vi "Scan Larvae Contour (SubVI).vi"(0 "Data In":u8=255, 1 "Input Valid?":bool, 3 "X Start":u16, 4 "Y Start":u16, 6 "Max. Scan Cycles":u32=40000) -> (13 "Ready for Input?":bool, 14 "Boundary Point XY":u32, 15 "Boundary Valid?":bool, 16 "Scan End?":bool, 19 "Total ClkCyls":u32)   [LabVIEW 2015]
uses:
  Controls (FPGA)/Larvae Contour States DRAM.ctl
  Controls (FPGA)/Contour Scan.ctl
  <vilib>/rvi/Emulation/niFpgaProcessEmulError.vi
  <vilib>/rvi/Emulation/niFpgaEmulationIsFPGAContextNoSignature.vi
  <vilib>/rvi/Emulation/niFpgaSctlEmulationGetInTimedLoop.vi
  <vilib>/rvi/errors/niFpgaSetErrorForExecOnDevCompSimple.vi
  <vilib>/rvi/eio/common/nirviEmuReportErrorAndStop.vi
  <vilib>/rvi/DataTransferAndStorage/Container/Common/niFpgaContainerGetUniqueNameForEmu.vi
  <vilib>/rvi/FIFO/Fifo_Resource/nirvififoEmulationSetSize.vi
  <vilib>/rvi/FIFO/Fifo_Resource/nirviFifoEmulationQueueMgr.vi
  <instcachedir>/0/nirviFifoEmulationQueueMgr_E5CAEC123FF24DC58D834DCA3CDAA9B5.lvgen/nirviFifoEmulationQueueMgr_E5CAEC123FF24DC58D834DCA3CDAA9B5_001.vi
  <vilib>/Utility/error.llb/Clear Errors.vi
  <vilib>/rvi/FIFO/Fifo_Resource/nirvififoEmulationCreateLock.vi
  <vilib>/rvi/FIFO/Fifo_Resource/nirvififoEmulationObtainLock.vi
  <vilib>/rvi/FIFO/Fifo_Resource/nirvififoEmulationReleaseLock.vi
  <vilib>/rvi/occurrence/nirviWaitOnOccurrenceBase.vi
  <vilib>/rvi/errors/nirviReportUnexpectedCaseInternalError.vi
  <vilib>/rvi/errors/nirviReportUnexpectedCaseInternalError (U32).vi
  <instcachedir>/0/nirviFifoEmulationQueueMgr_E5CAEC123FF24DC58D834DCA3CDAA9B5.lvgen/nirviFifoEmulationQueueMgr_E5CAEC123FF24DC58D834DCA3CDAA9B5_004.vi
  <vilib>/rvi/FIFO/Fifo_Resource/nirvififoEmulationDetermineInputValidOut.vi
  <vilib>/rvi/DataTransferAndStorage/Container/XNode/niFpgaContainer.xnode
  <vilib>/rvi/FIFO/Fifo_Resource/nirvififoEmulationRead.vi
  <vilib>/rvi/FIFO/Fifo_Resource/nirvififoEmulationWrite.vi
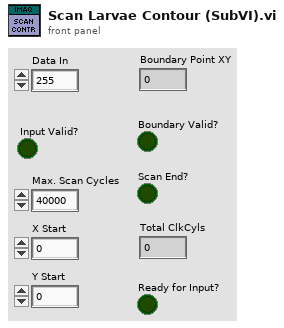
[diagram p1: front panel]
types:
  T1 = typedef "Contour Scan.ctl" = cluster{"Next Address":fxp<+,24,24>, "Next X":fxp<+,12,12>, "Next Y":fxp<+,12,12>, "Current Address":fxp<+,24,24>, "Current X":fxp<+,12,12>, "Current Y":fxp<+,12,12>, "Scan Count":u32}
  T2 = typedef "Larvae Contour States DRAM.ctl" = enum8{"Intialize", "Loop Condition", "Pixel 1", "Pixel 2", "Pixel 3", "Pixel 4", "Pixel 5", "Pixel 6", "Pixel 7", "Pixel 8", "Retrieve Data", "End of Scan"}
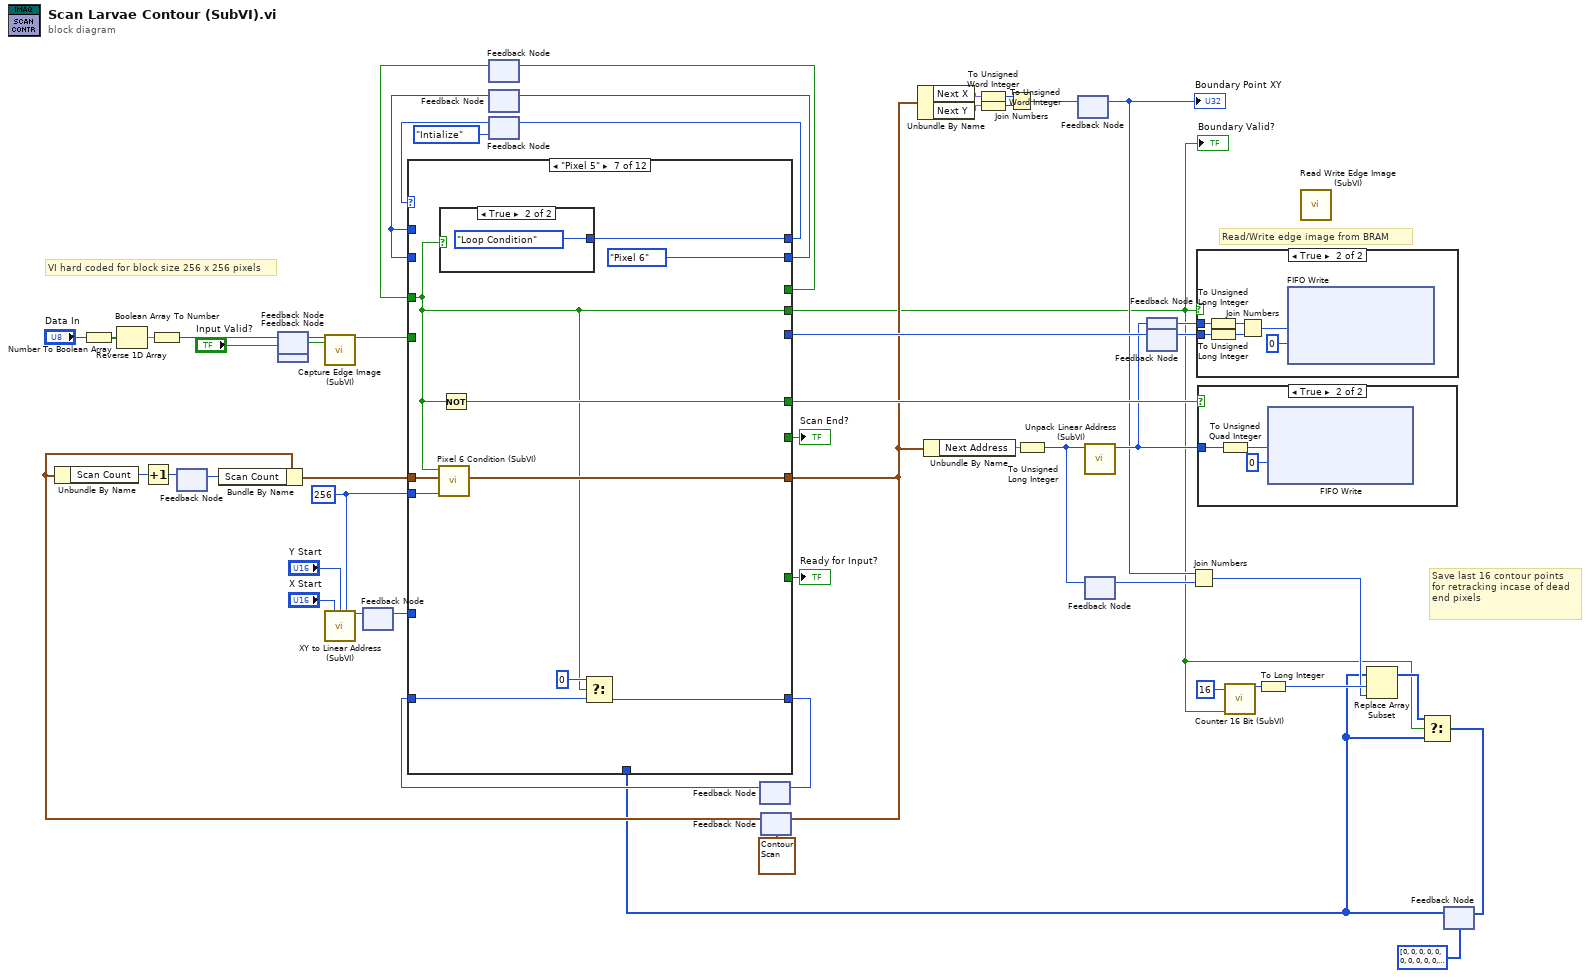
[diagram p0: block diagram]
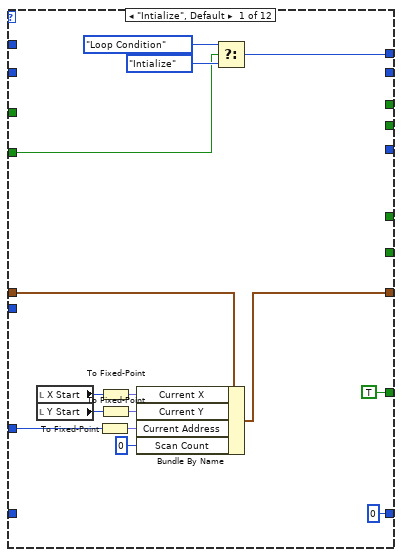
[diagram p4: hidden frame]
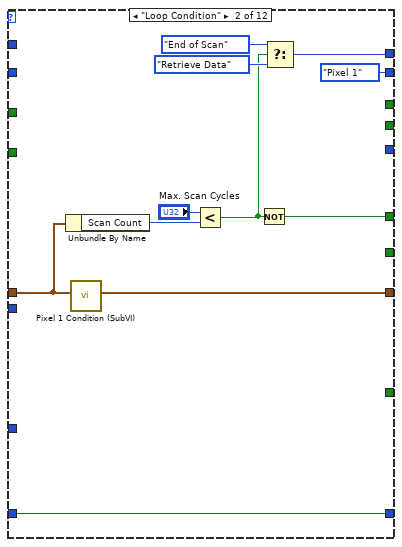
[diagram p5: hidden frame]
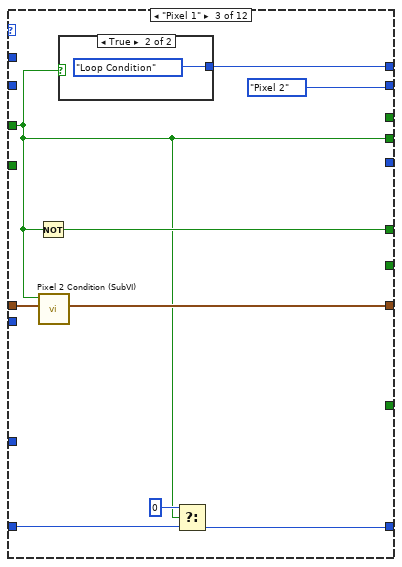
[diagram p6: hidden frame]
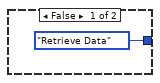
[diagram p7: hidden frame]
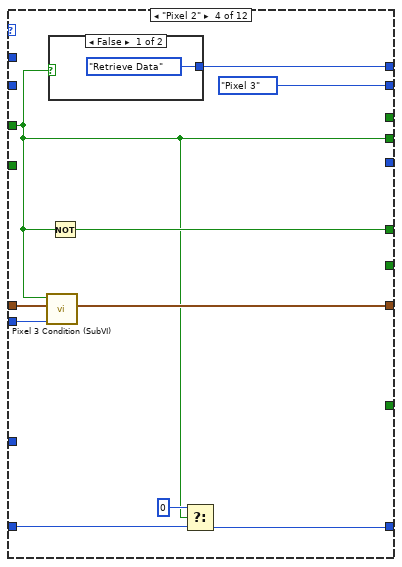
[diagram p8: hidden frame]
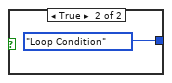
[diagram p9: hidden frame]
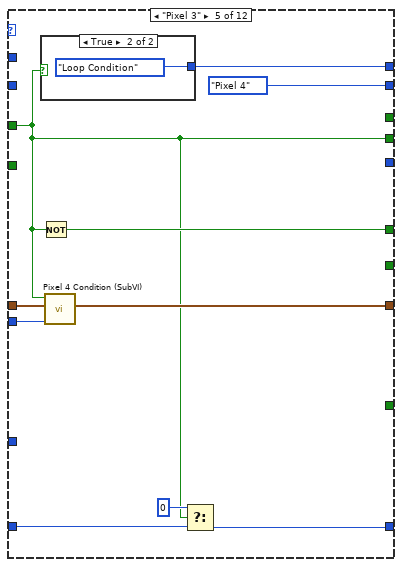
[diagram p10: hidden frame]
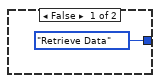
[diagram p11: hidden frame]
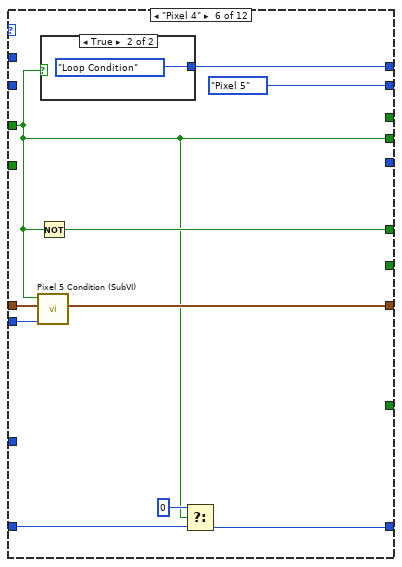
[diagram p12: hidden frame]
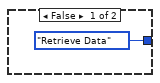
[diagram p13: hidden frame]
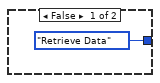
[diagram p14: hidden frame]
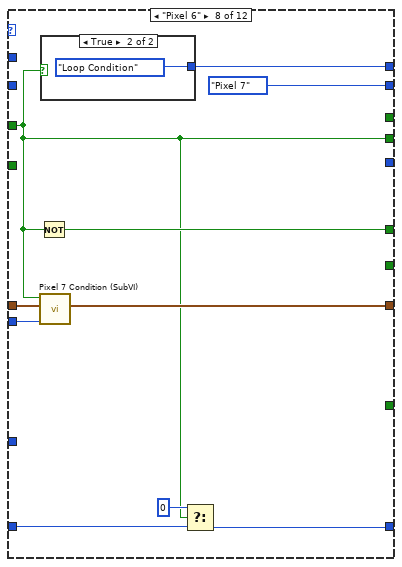
[diagram p15: hidden frame]
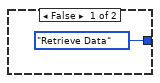
[diagram p16: hidden frame]
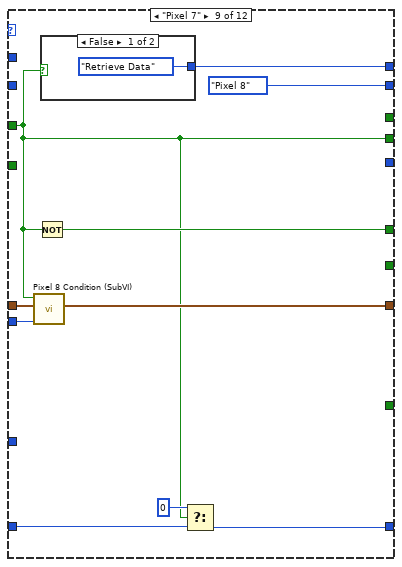
[diagram p17: hidden frame]
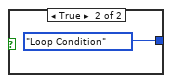
[diagram p18: hidden frame]
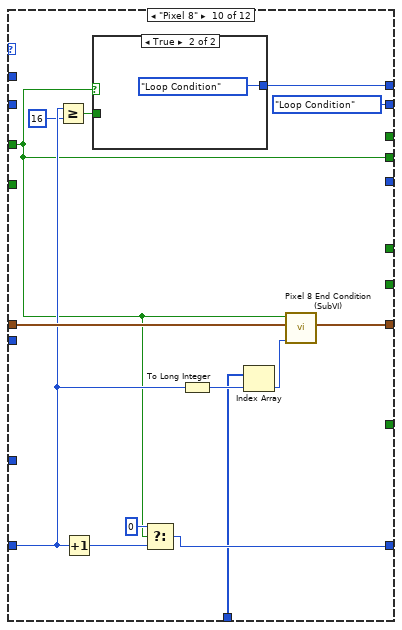
[diagram p19: hidden frame]
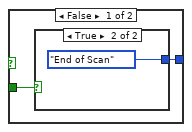
[diagram p20: hidden frame]
diagram:
  w23 = u16 256 ("Image Width")
  # "Save last 16 contour points for retracking incase of dead end pixels"
  # "VI hard coded for block size 256 x 256 pixels"
  # "Read/Write edge image from BRAM"
  n1 = Number To Boolean Array(number="Data In") -> (Boolean array=w21:bool[])
  n2 = Reverse 1D Array(array=w21) -> (reversed array=w22:bool[])
  n3 = Boolean Array To Number(Boolean array=w22) -> (number=w19:u8)
  n4 = feedback #1() -> (w30:u32)  [unwired: 1 in]
  n5 = feedback-in #2(w19) -> ()
  n6 = feedback #2() -> (w44:u8)  [unwired: 1 in]
  n7 = feedback-in #3("Input Valid?") -> ()
  n8 = feedback #3() -> (w43:bool)  [unwired: 1 in]
  n9 = call "Capture Edge Image (SubVI).vi"("Data In"=w44, "Data Valid?"=w43) -> ("Capture End?"=w42:bool)  [unwired: 17 in]
  n10 = call "XY to Linear Address (SubVI).vi"("X"="X Start", "Y"="Y Start", "Image Width"=w23) -> ("Linear Address"=w41:u32)  [unwired: 12 in]
  n11 = feedback-in #4(w41) -> ()
  n12 = feedback #4() -> (w40:u32)  [unwired: 1 in]
  n13 = feedback #5() -> (w17:bool)  [unwired: 1 in]
  n14 = feedback #6() -> (w50:T2)  [unwired: 1 in]
  n15 = feedback #7(Larvae_Contour_States_DRAM."Intialize") -> (w52:T2)
  n16 = feedback #8() -> (w12:u8)  [unwired: 1 in]
  n17 = feedback #9(T1 {"Next Address"=0.0, "Next X"=0.0, "Next Y"=0.0, "Current Address"=0.0, "Current X"=0.0, "Current Y"=0.0, "Scan Count"=0}) -> (w36:T1)
  n18 = Unbundle By Name(w36) -> ("Scan Count"=w35:u32)
  n19 = Increment(x=w35) -> (x+1=w34:u32)
  n20 = feedback-in #1(w34) -> ()
  n21 = Bundle By Name(cluster=w36, "Scan Count"=w30) -> (w37:T1)
  n22 = feedback #10() -> (w2:u32)  [unwired: 1 in]
  "Boundary Point XY" <- w2
  n23 = feedback #11() -> (w3:u32)  [unwired: 1 in]
  n24 = feedback #12() -> (w47:u32)  [unwired: 1 in]
  n25 = feedback #13() -> (w48:u8)  [unwired: 1 in]
  n26 = Join Numbers(hi=w2, lo=w3) -> ((hi.lo)=w8:u64)
  n27 = call "Read Write Edge Image (SubVI).vi"() -> ()  [unwired: 12 in]
  n28 = feedback #14(u64[] [0, 0, 0, 0, 0, 0, 0, 0, 0, 0, 0, 0, 0, 0, 0, 0]) -> (w6:u64[])
  n29 = case shown="\"Pixel 5\"" w52 {
    tunnel: [w68 w80 w89 w99 w111 w123 w135 w147 w159 w176 w198 Larvae_Contour_States_DRAM."Intialize" ("f")] -> w54
    tunnel: [_ _ w81 w92 w104 w116 w128 w140 w152 w166 _ _] -> w1
    tunnel: [_ _ _ _ _ _ _ _ _ _ _ TRUE] -> w27
    tunnel: w17 -> [_ _ w81 w92 w104 w116 w128 w140 w152 w166 _ _]
    tunnel: [_ w76 w88 w101 w113 w125 w137 w149 w161 _ _ _] -> w46
    tunnel: [_ Larvae_Contour_States_DRAM."Pixel 1" ("f") Larvae_Contour_States_DRAM."Pixel 2" ("f") Larvae_Contour_States_DRAM."Pixel 3" ("f") Larvae_Contour_States_DRAM."Pixel 4" ("f") Larvae_Contour_States_DRAM."Pixel 5" ("f") Larvae_Contour_States_DRAM."Pixel 6" ("f") Larvae_Contour_States_DRAM."Pixel 7" ("f") Larvae_Contour_States_DRAM."Pixel 8" ("f") Larvae_Contour_States_DRAM."Loop Condition" ("f") w197 _] -> w51
    tunnel: w50 -> [_ _ _ _ _ _ _ _ _ _ w199 _]
    tunnel: [_ _ _ _ _ _ _ _ _ _ w201 _] -> w5
    tunnel: w50 -> [_ _ _ _ _ _ _ _ _ _ w197 _]
    tunnel: [_ _ _ _ _ _ _ _ _ _ w193 _] -> w49
    tunnel: w42 -> [w66 _ _ _ _ _ _ _ _ _ _ _]
    tunnel: w40 -> [w64 _ _ _ _ _ _ _ _ _ _ _]
    tunnel: w37 -> [w65 w72 w86 w98 w109 w122 w134 w146 w157 w175 w186 w204]
    tunnel: [w62 w75 w85 w97 w110 w121 w133 w145 w158 w174 w186 w204] -> w26
    tunnel: w23 -> [_ _ _ w96 w108 w120 w132 w144 w156 _ _ _]
    tunnel: [TRUE _ _ _ _ _ _ _ _ _ _ _] -> w18
    tunnel: w6 -> [_ _ _ _ _ _ _ _ _ w164 _ _]
    tunnel: [u8 0 ("Scan Count") w70 w83 w94 w106 w118 w130 w142 w154 w171 w183 w202] -> w13
    tunnel: w12 -> [_ w70 w84 w95 w107 w119 w131 w143 w155 w169 w183 w202]
    frame "Intialize", Default {
      n30 = local read "X Start"() -> (w58:u16)
      n31 = local read "Y Start"() -> (w57:u16)
      n32 = To Fixed-Point(number=w64) -> (fixed-point=w59:fxp<+,24,24>)  [unwired: 1 in]
      n33 = To Fixed-Point(number=w58) -> (fixed-point=w61:fxp<+,12,12>)  [unwired: 1 in]
      n34 = To Fixed-Point(number=w57) -> (fixed-point=w60:fxp<+,12,12>)  [unwired: 1 in]
      n35 = Bundle By Name(cluster=w65, "Current X"=w61, "Current Y"=w60, "Current Address"=w59, "Scan Count"=u32 0) -> (w62:T1)
      n36 = Select(t=Larvae_Contour_States_DRAM."Loop Condition", s=w66, f=Larvae_Contour_States_DRAM."Intialize") -> (s? t:f=w68:T2)
    }
    frame "Loop Condition" {
      n37 = Unbundle By Name(w72) -> ("Scan Count"=w74:u32)
      n38 = call "Pixel 1 Condition (SubVI).vi"("Contour Scan in"=w72) -> ("Contour Scan out"=w75:T1)  [unwired: 10 in]
      n39 = Less?(x="Max. Scan Cycles", y=w74) -> (x < y?=w73:bool)
      n40 = Not(x=w73) -> (.not. x?=w76:bool)
      n41 = Select(t=Larvae_Contour_States_DRAM."End of Scan", s=w73, f=Larvae_Contour_States_DRAM."Retrieve Data") -> (s? t:f=w80:T2)
    }
    frame "Pixel 1" {
      n42 = Not(x=w81) -> (.not. x?=w88:bool)
      n43 = call "Pixel 2 Condition (SubVI).vi"("Contour Scan in"=w86, "Fnd?"=w81) -> ("Contour Scan out"=w85:T1)  [unwired: 9 in]
      n44 = case shown="True" w81 {
        tunnel: [Larvae_Contour_States_DRAM."Retrieve Data" ("f") Larvae_Contour_States_DRAM."Loop Condition" ("f")] -> w89
        frame False {
        }
        frame True {
        }
      }
      n45 = Select(t=u8 0, s=w81, f=w84) -> (s? t:f=w83:u8)
    }
    frame "Pixel 2" {
      n46 = call "Pixel 3 Condition (SubVI).vi"("Image Width"=w96, "Contour Scan in"=w98, "Fnd?"=w92) -> ("Contour Scan out"=w97:T1)  [unwired: 8 in]
      n47 = case shown="False" w92 {
        tunnel: [Larvae_Contour_States_DRAM."Retrieve Data" ("f") Larvae_Contour_States_DRAM."Loop Condition" ("f")] -> w99
        frame False {
        }
        frame True {
        }
      }
      n48 = Not(x=w92) -> (.not. x?=w101:bool)
      n49 = Select(t=u8 0, s=w92, f=w95) -> (s? t:f=w94:u8)
    }
    frame "Pixel 3" {
      n50 = case shown="True" w104 {
        tunnel: [Larvae_Contour_States_DRAM."Retrieve Data" ("f") Larvae_Contour_States_DRAM."Loop Condition" ("f")] -> w111
        frame False {
        }
        frame True {
        }
      }
      n51 = Not(x=w104) -> (.not. x?=w113:bool)
      n52 = call "Pixel 4 Condition (SubVI).vi"("Image Width"=w108, "Contour Scan in"=w109, "Fnd?"=w104) -> ("Contour Scan out"=w110:T1)  [unwired: 8 in]
      n53 = Select(t=u8 0, s=w104, f=w107) -> (s? t:f=w106:u8)
    }
    frame "Pixel 4" {
      n54 = call "Pixel 5 Condition (SubVI).vi"("Image Width"=w120, "Contour Scan in"=w122, "Fnd?"=w116) -> ("Contour Scan out"=w121:T1)  [unwired: 8 in]
      n55 = Not(x=w116) -> (.not. x?=w125:bool)
      n56 = case shown="True" w116 {
        tunnel: [Larvae_Contour_States_DRAM."Retrieve Data" ("f") Larvae_Contour_States_DRAM."Loop Condition" ("f")] -> w123
        frame False {
        }
        frame True {
        }
      }
      n57 = Select(t=u8 0, s=w116, f=w119) -> (s? t:f=w118:u8)
    }
    frame "Pixel 5" {
      n58 = call "Pixel 6 Condition (SubVI).vi"("Image Width"=w132, "Contour Scan in"=w134, "Fnd?"=w128) -> ("Contour Scan out"=w133:T1)  [unwired: 8 in]
      n59 = case shown="True" w128 {
        tunnel: [Larvae_Contour_States_DRAM."Retrieve Data" ("f") Larvae_Contour_States_DRAM."Loop Condition" ("f")] -> w135
        frame False {
        }
        frame True {
        }
      }
      n60 = Not(x=w128) -> (.not. x?=w137:bool)
      n61 = Select(t=u8 0, s=w128, f=w131) -> (s? t:f=w130:u8)
    }
    frame "Pixel 6" {
      n62 = Not(x=w140) -> (.not. x?=w149:bool)
      n63 = call "Pixel 7 Condition (SubVI).vi"("Image Width"=w144, "Contour Scan in"=w146, "Fnd?"=w140) -> ("Contour Scan out"=w145:T1)  [unwired: 8 in]
      n64 = case shown="True" w140 {
        tunnel: [Larvae_Contour_States_DRAM."Retrieve Data" ("f") Larvae_Contour_States_DRAM."Loop Condition" ("f")] -> w147
        frame False {
        }
        frame True {
        }
      }
      n65 = Select(t=u8 0, s=w140, f=w143) -> (s? t:f=w142:u8)
    }
    frame "Pixel 7" {
      n66 = call "Pixel 8 Condition (SubVI).vi"("Image Width"=w156, "Contour Scan in"=w157, "Fnd?"=w152) -> ("Contour Scan out"=w158:T1)  [unwired: 8 in]
      n67 = Not(x=w152) -> (.not. x?=w161:bool)
      n68 = case shown="False" w152 {
        tunnel: [Larvae_Contour_States_DRAM."Retrieve Data" ("f") Larvae_Contour_States_DRAM."Loop Condition" ("f")] -> w159
        frame False {
        }
        frame True {
        }
      }
      n69 = Select(t=u8 0, s=w152, f=w155) -> (s? t:f=w154:u8)
    }
    frame "Pixel 8" {
      n70 = Greater Or Equal?(x=w169, y=u8 16) -> (x >= y?=w167:bool)
      n71 = Increment(x=w169) -> (x+1=w170:u8)
      n72 = case shown="True" w166 {
        tunnel: [w179 Larvae_Contour_States_DRAM."Loop Condition" ("f")] -> w176
        tunnel: w167 -> [w178 _]
        frame False {
          n73 = case shown="True" w178 {
            tunnel: [Larvae_Contour_States_DRAM."Loop Condition" ("f") Larvae_Contour_States_DRAM."End of Scan" ("f")] -> w179
            frame False {
            }
            frame True {
            }
          }
        }
        frame True {
        }
      }
      n74 = Select(t=u8 0, s=w166, f=w170) -> (s? t:f=w171:u8)
      n75 = To Long Integer(number=w169) -> (32bit integer=w172:i32)
      n76 = Index Array(array=w164, index=w172) -> (element=w165:u64)
      n77 = call "Pixel 8 End Condition (SubVI).vi"("Previous Fnd Location"=w165, "Contour Scan in"=w175, "Fnd?"=w166) -> ("Contour Scan out"=w174:T1)  [unwired: 8 in]
    }
    frame "Retrieve Data" {
      n78 = xnode ("FIFO Write")("Timeout"=0) -> ("Element"=w190:u8, "Timed Out?"=w191:bool)  [unwired: 1 in, 1 out]
      n79 = Unbundle By Name(w186) -> ("Next Address"=w185:fxp<+,24,24>)
      n80 = To Unsigned Long Integer(number=w185) -> (unsigned 32bit integer=w184:u32)
      n81 = Not(x=w191) -> (.not. x?=w189:bool)
      n82 = call "Unpack Linear Address (SubVI).vi"("Linear Address"=w184) -> ("Bit Address"=w187:u8)  [unwired: 9 in, 1 out]
      n83 = Select(t=w199, s=w189, f=Larvae_Contour_States_DRAM."Retrieve Data") -> (s? t:f=w198:T2)
      n84 = Number To Boolean Array(number=w190) -> (Boolean array=w194:bool[])
      n85 = To Long Integer(number=w187) -> (32bit integer=w188:i32)
      n86 = Replace Array Subset(array=w194, new element=FALSE ("new element/subarray"), index=w188) -> (w196:bool[])
      n87 = Index Array(array=w194, index=w188) -> (element=w201:bool)
      n88 = Boolean Array To Number(Boolean array=w196) -> (number=w193:u8)
    }
    frame "End of Scan" {
      n89 = Unbundle By Name(w204) -> ("Scan Count"=→"Total ClkCyls":u32)
    }
  }
  "Scan End?" <- w27
  "Boundary Valid?" <- w1
  "Ready for Input?" <- w18
  n90 = feedback-in #5(w5) -> ()
  n91 = feedback-in #6(w51) -> ()
  n92 = feedback-in #7(w54) -> ()
  n93 = feedback-in #8(w13) -> ()
  n94 = feedback-in #9(w26) -> ()
  n95 = Unbundle By Name(w26) -> ("Next X"=w33:fxp<+,12,12>, "Next Y"=w32:fxp<+,12,12>)
  n96 = Unbundle By Name(w26) -> ("Next Address"=w31:fxp<+,24,24>)
  n97 = To Unsigned Word Integer(number=w33) -> (unsigned 16bit integer=w29:u16)
  n98 = To Unsigned Word Integer(number=w32) -> (unsigned 16bit integer=w28:u16)
  n99 = Join Numbers(hi=w29, lo=w28) -> ((hi.lo)=w14:u32)
  n100 = To Unsigned Long Integer(number=w31) -> (unsigned 32bit integer=w4:u32)
  n101 = feedback-in #10(w14) -> ()
  n102 = call "Unpack Linear Address (SubVI).vi"("Linear Address"=w4) -> ("Packet Address"=w39:u32)  [unwired: 9 in, 1 out]
  n103 = feedback-in #11(w4) -> ()
  n104 = feedback-in #12(w39) -> ()
  n105 = feedback-in #13(w49) -> ()
  n106 = case shown="True" w1 {
    tunnel: w48 -> [_ w212]
    tunnel: w47 -> [_ w207]
    frame False {
    }
    frame True {
      n107 = To Unsigned Long Integer(number=w207) -> (unsigned 32bit integer=w210:u32)
      n108 = To Unsigned Long Integer(number=w212) -> (unsigned 32bit integer=w211:u32)
      n109 = Join Numbers(hi=w210, lo=w211) -> ((hi.lo)=w209:u64)
      n110 = xnode ("FIFO Write")("Element"=w209, "Timeout"=0) -> ()  [unwired: 1 in, 2 out]
    }
  }
  n111 = case shown="True" w46 {
    tunnel: w39 -> [_ w214]
    frame False {
    }
    frame True {
      n112 = To Unsigned Quad Integer(1:w214) -> (0:w213:u64)
      n113 = xnode ("FIFO Write")("Element"=w213, "Timeout"=0) -> ()  [unwired: 1 in, 2 out]
    }
  }
  n114 = call "Counter 16 Bit (SubVI).vi"("Max. Count"=u16 16, "Enable"=w1) -> ("Count"=w10:u16)  [unwired: 11 in, 2 out]
  n115 = To Long Integer(number=w10) -> (32bit integer=w9:i32)
  n116 = Replace Array Subset(array=w6, new element=w8, index=w9) -> (w16:u64[])
  n117 = Select(t=w16, s=w1, f=w6) -> (s? t:f=w7:u64[])
  n118 = feedback-in #14(w7) -> ()
